vi "Get_Latest_Build_From_Artifactory.vi"(7 "Repository":string="CIBuild_2015", 11 "Error In":errorcluster) -> (4 "Output Path":path, 15 "Error Out 2":errorcluster)   [LabVIEW 2016, in "2015 VA Washer.lvlib"]
uses:
  Projects/2015 VA Washer.lvlib
  <vilib>/regexp/Match Regular Expression.xnode
  <vilib>/httpClient/LabVIEWHTTPClient.lvlib
  <vilib>/zip/NI_Unzip.lvlib
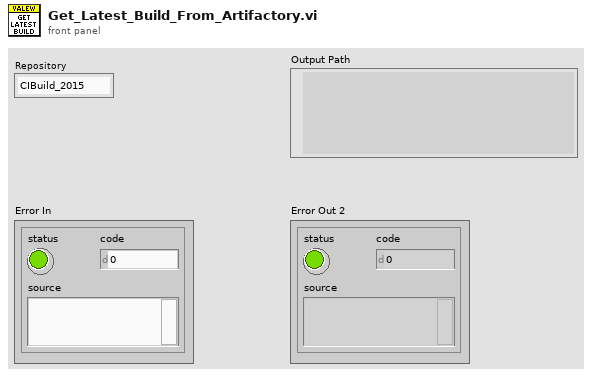
[diagram p1: front panel]
types:
  T1 = typedef "LabVIEWHTTPClient.lvlib/ClientHandle.ctl" = refnum<k1>
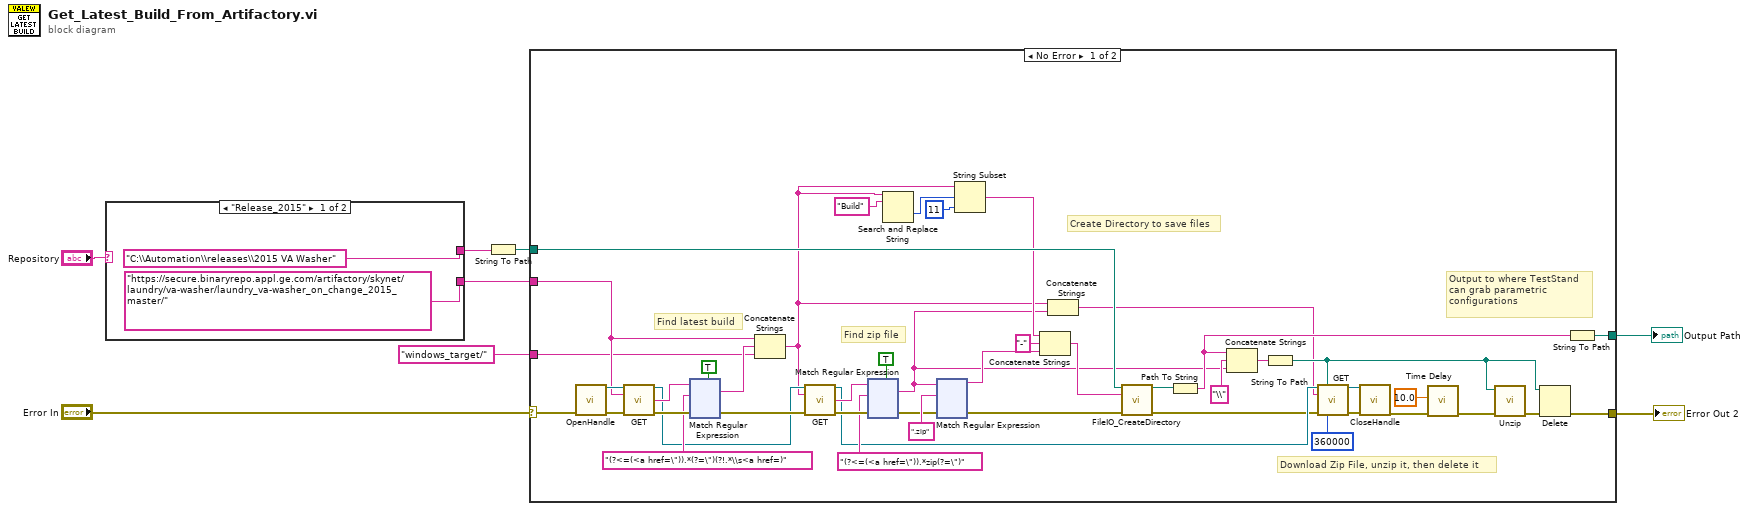
[diagram p0: block diagram]
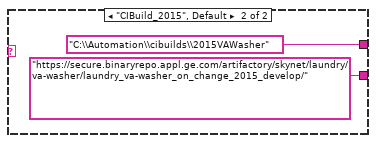
[diagram p2: hidden frame]
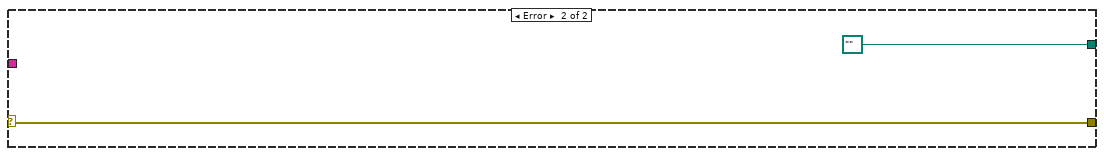
[diagram p3: hidden frame]
diagram:
  n1 = case shown="\"Release_2015\"" "Repository" {
    tunnel: ["C:\\Automation\\releases\\2015 VA Washer" "C:\\Automation\\cibuilds\\2015VAWasher"] -> w5
    tunnel: ["https://secure.binaryrepo.appl.ge.com/artifactory/skynet/laundry/va-washer/laundry_va-washer_on_change_2015_master/" "https://secure.binaryrepo.appl.ge.com/artifactory/skynet/laundry/va-washer/laundry_va-washer_on_change_2015_develop/"] -> w2
    frame "Release_2015" {
    }
    frame "CIBuild_2015", Default {
    }
  }
  n2 = String To Path(string=w5) -> (path=w4:path)
  n3 = case shown="No Error" "Error In" {
    selector: "Error In" -> [w56 w402]
    tunnel: [w35 w402] -> w6
    tunnel: [w30 path ""] -> w7
    tunnel: w4 -> [w31 _]
    tunnel: w2 -> [w27 _]
    tunnel: "windows_target/" -> [w26 _]
    frame No Error {
      # "Create Directory to save files"
      # "Output to where TestStand\ncan grab parametric\nconfigurations"
      # "Find zip file"
      # "Find latest build"
      # "Download Zip File, unzip it, then delete it"
      n4 = call <vilib>:"OpenHandle.vi"("error in (no error)"=w56) -> ("client handle out"=w57:T1, "error out"=w58:errorcluster)  [unwired: 13 in]
      n5 = call <vilib>:"GET.vi"("client handle"=w57, "url"=w27, "error in (no error)"=w58) -> ("client handle out"=w49:T1, "body"=w54:string, "error out"=w55:errorcluster)  [unwired: 9 in, 1 out]
      n6 = xnode "Match Regular Expression"("input string"=w54, "regular expression"="(?<=(<a href=\")).*(?=\")(?!.*\\s<a href=)", "error in"=w55, "multiline? (F)"=TRUE) -> ("whole match"=w53:string, "error out"=w50:errorcluster)  [unwired: 2 in, 3 out]
      n7 = Concatenate Strings(w27, w53, w26) -> (w18:string)
      n8 = call <vilib>:"GET.vi"("client handle"=w49, "url"=w18, "error in (no error)"=w50) -> ("client handle out"=w42:T1, "body"=w46:string, "error out"=w47:errorcluster)  [unwired: 9 in, 1 out]
      n9 = xnode "Match Regular Expression"("input string"=w46, "regular expression"="(?<=(<a href=\")).*zip(?=\")", "error in"=w47, "multiline? (F)"=TRUE) -> ("whole match"=w17:string, "error out"=w39:errorcluster)  [unwired: 2 in, 3 out]
      n10 = Search and Replace String(input string=w18, search string="Build") -> (offset past replacement=w23:i32)  [unwired: 6 in, 3 out]
      n11 = xnode "Match Regular Expression"("input string"=w17, "regular expression"=".zip", "error in"=w39) -> ("before match"=w20:string, "error out"=w38:errorcluster)  [unwired: 3 in, 3 out]
      n12 = String Subset(string=w18, offset (0)=w23, length (rest)=11 ("length (rest)")) -> (substring=w21:string)
      n13 = Concatenate Strings(w21, "-" ("string"), w20) -> (w19:string)
      n14 = Concatenate Strings(w18, w17) -> (w16:string)
      n15 = call "FileIO_CreateDirectory.vi"("Base Path"=w31, "Directory Name"=w19, "Error In"=w38) -> ("File Path Control"=w34:path, "Error Out"=w41:errorcluster)  [unwired: 11 in]
      n16 = Path To String(path=w34) -> (string=w28:string)
      n17 = Concatenate Strings(w28, "\\" ("string"), w17) -> (w36:string)
      n18 = String To Path(string=w36) -> (path=w33:path)
      n19 = call <vilib>:"GET.vi"("client handle"=w42, "output file"=w33, "url"=w16, "error in (no error)"=w41, "timeout (10000)"=360000) -> ("client handle out"=w44:T1, "error out"=w43:errorcluster)  [unwired: 7 in, 2 out]
      n20 = call <vilib>:"CloseHandle.vi"("client handle"=w44, "error in (no error)"=w43) -> ("error out"=w14:errorcluster)  [unwired: 13 in]
      n21 = call "Time Delay"("error in (no error)"=w14, "Delay Time (s)"=10.0) -> ("error out"=w13:errorcluster)  [unwired: 9 in]
      n22 = call <vilib>:"Unzip.vi"("error in (no error)"=w13, "Zip file"=w33) -> ("error out"=w32:errorcluster)  [unwired: 7 in, 2 out]
      n23 = Delete(path (use dialog)=w33, error in=w32) -> (error out=w35:errorcluster)  [unwired: 3 in, 2 out]
      n24 = String To Path(string=w28) -> (path=w30:path)
    }
    frame Error {
    }
  }
  "Output Path" <- w7
  "Error Out 2" <- w6
